vi "Example Output.vi"() -> ()   [LabVIEW 2015]
uses:
  Output/Output.lvclass
  Request/Request.lvclass
panel:
  in  "Answer":string="Greetings Back!"
  out "Greeting":string
  out "error out":errorcluster
  in  "Stop Button":bool
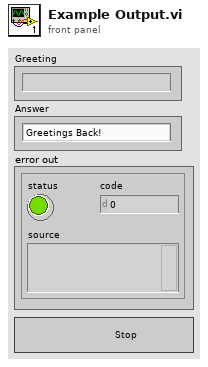
[diagram p1: front panel]
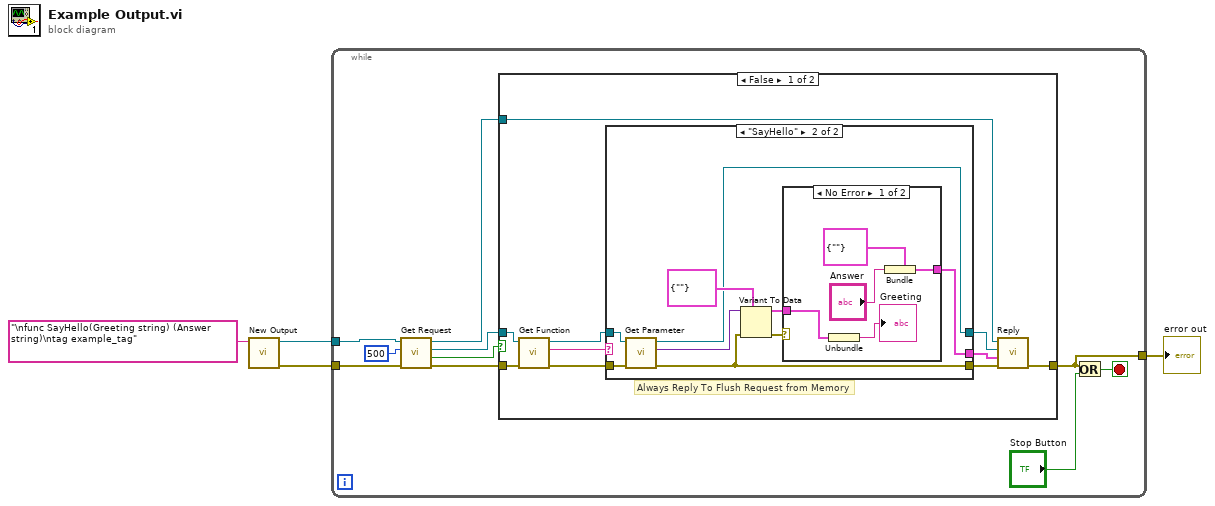
[diagram p0: block diagram]
diagram:
  n1 = call "New Output.vi"("Descriptor"="\nfunc SayHello(Greeting string) (Answer string)\ntag example_tag") -> ("error out"=w2:errorcluster, "output"=w3:refnum<class "Output.lvclass">)  [unwired: 9 in]
  n2 = while {
    tunnel: w3 -> [w14]
    tunnel: w2 -> [w9]
    tunnel: [w5] -> w1
    stop <- w7 stop-if-true
    n3 = call "Get Request.vi"("error in (no error)"=w9, "timeout in ms (-1)"=500, "output in"=w14) -> ("error out"=w8:errorcluster, "timed out?"=w12:bool, "request.lvclass"=w11:refnum<class "Request.lvclass">, "output out"=w10:refnum<class "Output.lvclass">)  [unwired: 5 in]
    n4 = case shown="False" w12 {
      tunnel: w11 -> [w24 _]
      tunnel: w10 -> [w22 _]
      tunnel: w8 -> [w18 w41]
      tunnel: [w15 w41] -> w5
      frame False {
        # "Always Reply To Flush Request from Memory"
        n5 = call "Get Function.vi"("error in (no error)"=w18, "request in"=w24) -> ("error out"=w17:errorcluster, "function"=w23:string, "request out"=w21:refnum<class "Request.lvclass">)  [unwired: 7 in]
        n6 = case shown="\"SayHello\"" w23 {
          tunnel: w21 -> [w26 w35]
          tunnel: [w26 w30] -> w20
          tunnel: [_ w31] -> w19
          tunnel: w17 -> [w25 w28]
          tunnel: [w25 w27] -> w16
          frame "False", Default {
          }
          frame "SayHello" {
            n7 = call "Get Parameter.vi"("error in (no error)"=w28, "request in"=w35) -> ("error out"=w27:errorcluster, "parameter"=w33:variant, "request out"=w30:refnum<class "Request.lvclass">)  [unwired: 7 in]
            n8 = Variant To Data(error in=w27, type=cluster{"Greeting":string} {"Greeting"=""}, Variant=w33) -> (data=w32:cluster{"Greeting":string}, error out=w29:errorcluster)
            n9 = case shown="No Error" w29 {
              tunnel: w32 -> [w40 _]
              tunnel: [w37 _] -> w31
              frame No Error {
                n10 = Unbundle(w40) -> ("Greeting"=→"Greeting":string)
                n11 = Bundle(cluster=cluster{"Answer":string} {"Answer"=""}, "Answer"="Answer") -> (w37:cluster{"Answer":string})
              }
              frame Error {
              }
            }
          }
        }
        n12 = call "Reply.vi"("error in (no error)"=w16, "parameter"=w19, "request"=w20, "output in"=w22) -> ("error out"=w15:errorcluster)  [unwired: 6 in, 1 out]
      }
      frame True {
      }
    }
    n13 = Or(x=w5, y="Stop Button") -> (x .or. y?=w7:bool)
  }
  "error out" <- w1
